vi "Configure Measurement (Power State CCDF).vi"(0 "VISA resource name":refnum<visa-resource-name>, 5 "Measurement Bandwidth (5MHz)":dbl=5000000.0 format="%#.6g", 7 "Counts (100000)":dbl=100000.0 format="%#.6g", 9 "Measurement Interval (1ms)":dbl=0.001 format="%#.6g", 11 "error in (no error)":errorcluster) -> (4 "VISA resource name out":refnum<visa-resource-name>, 15 "error out":errorcluster)   [LabVIEW 2014, in "Agilent ESA PSA Series.lvlib"]
doc: "Sets up Power Complementary cumulative distribution function (CCDF) measurement operation."
uses:
  Agilent ESA PSA Series.lvlib
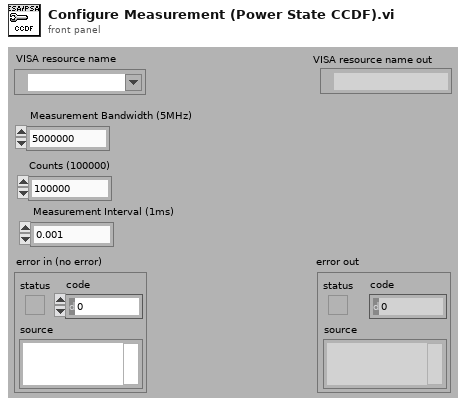
[diagram p1: front panel]
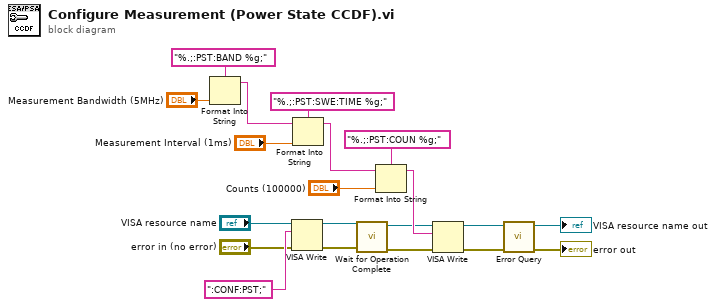
[diagram p0: block diagram]
diagram:
  n1 = Format Into String(format string="%.;:PST:BAND %g;", "Measurement Bandwidth (5MHz)") -> (resulting string=w16:string)  [unwired: 2 in, 1 out]
  n2 = VISA Write(VISA resource name="VISA resource name", write buffer=":CONF:PST;" ("initial string"), error in (no error)="error in (no error)") -> (VISA resource name out=w8:refnum<visa-resource-name>, error out=w9:errorcluster)  [unwired: 1 out]
  n3 = Format Into String(format string="%.;:PST:SWE:TIME %g;", initial string=w16, "Measurement Interval (1ms)") -> (resulting string=w13:string)  [unwired: 1 in, 1 out]
  n4 = call "Wait for Operation Complete.vi"("error in (no error)"=w9, "VISA resource name"=w8) -> ("error out"=w4:errorcluster, "VISA resource name out"=w5:refnum<visa-resource-name>)  [unwired: 8 in]
  n5 = Format Into String(format string="%.;:PST:COUN %g;", initial string=w13, "Counts (100000)") -> (resulting string=w10:string)  [unwired: 1 in, 1 out]
  n6 = VISA Write(VISA resource name=w5, write buffer=w10, error in (no error)=w4) -> (VISA resource name out=w6:refnum<visa-resource-name>, error out=w7:errorcluster)  [unwired: 1 out]
  n7 = call "Error Query.vi"("error in (no error)"=w7, "VISA resource name"=w6) -> ("error out"=→"error out":errorcluster, "VISA resource name out"=→"VISA resource name out":refnum<visa-resource-name>)  [unwired: 6 in, 2 out]
